vi "Get Count for Labels in Channel.vi"(8 "error in":errorcluster, 9 "labels settings for RT":T1[](array[typedef]) {"Label Timestamp Channel Data Reference" format="%.0x"; "Word Initial Raw Value" format="%032.0f"; "Label Disable/Trigger Channel Reference" format="%.0x"; "parameter driver data"."Tx parameter refs" format="%.0x"; "SDI" format="%02b"; "label" format="%.0o"}, 10 "channel number in":u8, 11 "board handle in":u8) -> (0 "error out":errorcluster, 1 "labels updated?":bool[](array[boolean]), 2 "channel number out":u8, 3 "board handle out":u8)   [LabVIEW 2020, in "AIM ARINC 429 Hardware API.lvlib"]
uses:
  AIM ARINC 429 Hardware API.lvlib
  <instrlib>/AIM GmbH/_ARINC-429/AIM429LV.lvlib
  Shared/Label.ctl
  <vilib>/NI/NI VeriStand Encoding and Decoding/Encoding.ctl
  <vilib>/NI/NI VeriStand Encoding and Decoding/Encoding and Decoding.lvlib
  Shared/Parameter Definition.ctl
  <vilib>/NI VeriStand/Custom Device API/Custom Device Item Ref.ctl
  <vilib>/NI VeriStand/Custom Device API/Custom Device API.lvlib
  Shared/RT Parameters.ctl
  Shared/Transfer Type.ctl
  <vilib>/NI VeriStand/Custom Device API/Data Reference.ctl
  Shared/RT Label Settings.ctl
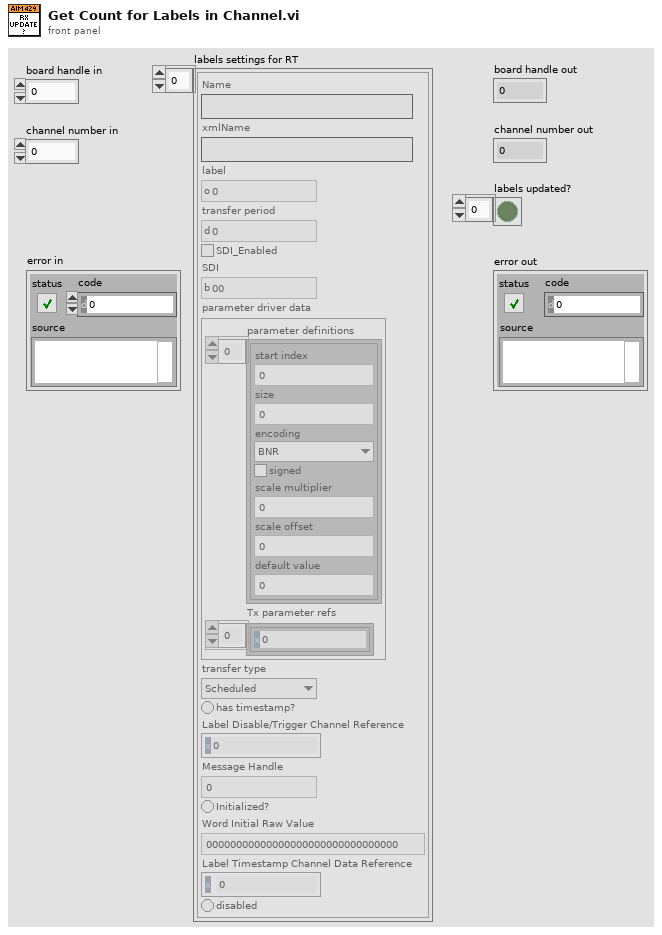
[diagram p1: front panel]
types:
  T1 = typedef "RT Label Settings.ctl" = cluster{"Name":string, "xmlName":string, "label":T2, "transfer period":u32, "SDI_Enabled":bool, "SDI":u8, "parameter driver data":T3, "transfer type":T7, "has timestamp?":bool, "Label Disable/Trigger Channel Reference":T6, "Message Handle":u64, "Initialized?":bool, "Word Initial Raw Value":u32, "Label Timestamp Channel Data Reference":T8, "disabled":bool}
  T2 = typedef "Label.ctl" = u8
  T3 = typedef "RT Parameters.ctl" = cluster{"parameter definitions":T4[], "Tx parameter refs":T6[]}
  T4 = typedef "Parameter Definition.ctl" = cluster{"start index":i32, "size":i32, "encoding":T5, "signed":bool, "scale multiplier":dbl, "scale offset":dbl, "default value":dbl}
  T5 = typedef "Encoding and Decoding.lvlib/Encoding.ctl" = enum16{"BNR", "BCD", "Discrete"}
  T6 = typedef "Custom Device API.lvlib/Custom Device Item Ref.ctl" = u64
  T7 = typedef "Transfer Type.ctl" = enum16{"Scheduled", "Acyclic", "Block", "Strobe"}
  T8 = typedef "Custom Device API.lvlib/Data Reference.ctl" = i32
  T9 = map{cluster{"board handle in":u8, "channel number in":u8, "label":T2, "SDI":u8}, i32}
  T10 = cluster{"board handle in":u8, "channel number in":u8, "label":T2, "SDI":u8}
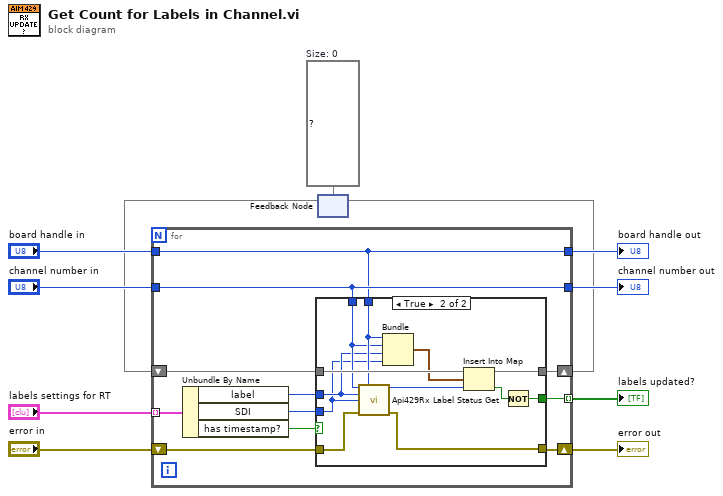
[diagram p0: block diagram]
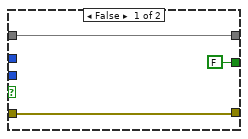
[diagram p2: hidden frame]
diagram:
  w4 = T9 {}  # Size: 0
  n1 = feedback #1(w4) -> (w3:T9)
  n2 = for {
    tunnel: "board handle in" -> [w16]
    tunnel: "channel number in" -> [w17]
    tunnel: "labels settings for RT" -> [w22] mode=indexing
    shift-right: [w18] -> w7
    shift-left: "error in" -> [w19]
    tunnel: [w17] -> w6
    tunnel: [w16] -> w5
    shift-right: [w13] -> w2
    shift-left: w3 -> [w14]
    tunnel: [w12] -> w1 mode=indexing
    n3 = Unbundle By Name(w22) -> ("label"=w21:T2, "SDI"=w20:u8, "has timestamp?"=w15:bool)
    n4 = case shown="True" w15 {
      tunnel: w21 -> [_ w31]
      tunnel: w20 -> [_ w30]
      tunnel: w19 -> [w25 w37]
      tunnel: [w25 w36] -> w18
      tunnel: w17 -> [_ w32]
      tunnel: w16 -> [_ w33]
      tunnel: w14 -> [w23 w34]
      tunnel: [w23 w28] -> w13
      tunnel: [FALSE w26] -> w12
      frame False {
      }
      frame True {
        n5 = call <instrlib>:"Api429Rx Label Status Get.vi"("b_Chn"=w32, "board_handle"=w33, "b_Label"=w31, "b_Sdi"=w30, "error in (no error)"=w37) -> ("px_LabCnt out"=w35:u32, "error out"=w36:errorcluster)  [unwired: 7 in, 2 out]
        n6 = Bundle("board handle in"=w33, "channel number in"=w32, "label"=w31, "SDI"=w30) -> (w29:T10)  [unwired: 1 in]
        n7 = Insert Into Map(map in=w34, key=w29, value=w35) -> (map out=w28:T9, value unchanged?=w27:bool)  [unwired: 1 out]
        n8 = Not(x=w27) -> (.not. x?=w26:bool)
      }
    }
  }
  "board handle out" <- w5
  "channel number out" <- w6
  "error out" <- w7
  "labels updated?" <- w1
  n9 = feedback-in #1(w2) -> ()
